vi "DetermineSetChosen.vi"(6 "Settings":T2={"Name of test"="", "Date"=timestamp(0 s since 1904-01-01), "Location"="", "Template"="", "Soundcard"="", "resolution"=32, "Sampling rate"=48000, "Ch1 Gain "=25.0, "Ch2 Gain"=10.0, "Sample time (s)"=0.3, "Pre-trigger (s)"=0.01, "Hammer Threshold"=10.0, "Positions"=12, "Taps/Position"=5, "Set Names"="", "Freq resolution"=10.0, "Hammer cutoff"=0.0, "Mic cutoff"=0.0, "Double bounce "=0.0, "Hammer Cal"=10.0, "dB Offset"=0.0, "Accel Cal"=10.0, "Vibrometer Cal"=0.0, "Mic Cal"=0.0, "Output"=2, "Voltage Cal"=1.0, "Vibrometer Port"="ASRL27::INSTR", "Range"=4, "High Pass"=2, "Bandwidth"=4, "X Range"=[], "Y Range"=[], "dB Spread"=0.0, "Trigger"=0, "Ch_1"=25, "Ch_2"=25, "flip?"=FALSE, "60Hz"=FALSE, "Time offset"=0.0, "Piezo Cal"=1.0, "Default Notes"=""} {"Ch_2" min=1 step=1; "Ch_1" min=1 max=100 step=1; "Trigger" items=["Hammer (force)", "Self-tap", "Spacebar"]; "Bandwidth" items=["1 kHz"=1, "5 kHz"=5, "10 kHz"=10, "25 kHz"=25, "50 kHz"=50, "100 kHz"=100]; "High Pass" items=["Off", "13 Hz", "104 Hz"]; "Range" items=["10 mm/s"=1, "20 mm/s"=2, "50 mm/s"=5, "100 mm/s"=10, "200 mm/s"=20, "500 mm/s"=50, "1 m/s"=100, "2 m/s"=200]; "Output" items=["Accelerometer", "Speed (from acceleration)", "Microphone", "Vibrometer", "Piezo"]; "Voltage Cal" format="%#_13g"; "Ch2 Gain" format="%#_13g"; "Ch1 Gain" format="%#_13g"; "Double bounce" min=0.0; "Mic cutoff" min=0.0 format="%#_4g"; "Hammer cutoff" min=0.0 format="%#_4g"; "Freq resolution" min=0.0; "Pre-trigger (s)" format="%#_13g"; "Date" format="%<%H:%M\n%d/%m/%y>T"; "resolution" items=["16 bit"=16, "24 bit"=24, "32 bit"=32]; "Sampling rate" items=["22050 samp/s"=22050, "44100 samp/s"=44100, "48000 samp/s"=48000]}, 9 "Bounds":T1, 11 "Mouse":T3) -> (1 "Queue Task":string, 3 "appended path":path)   [LabVIEW 2022 SP3]
uses:
  <vilib>/Utility/miscctls.llb/LVMouseTypeDef.ctl
  PreferencesControl.ctl
  <vilib>/Utility/miscctls.llb/LVBoundsTypeDef.ctl
  Mic/Mic_Global.vi
panel:
  in  "Cancel":bool
  in  "Just":bool
  in  "Subsequent":bool
  out "resulting string":string
  # "Hz"
  # "dB"
  # "dB"
  # "sec"
  # "sec"
  # "mV/Pa"
  # "mV/m/s2"
  # "mV/mm/s"
  # "V/N"
  # "sec"
  # "sec"
  # "mV/N"
  # "a.u."
  # "a.u."
  # "sec"
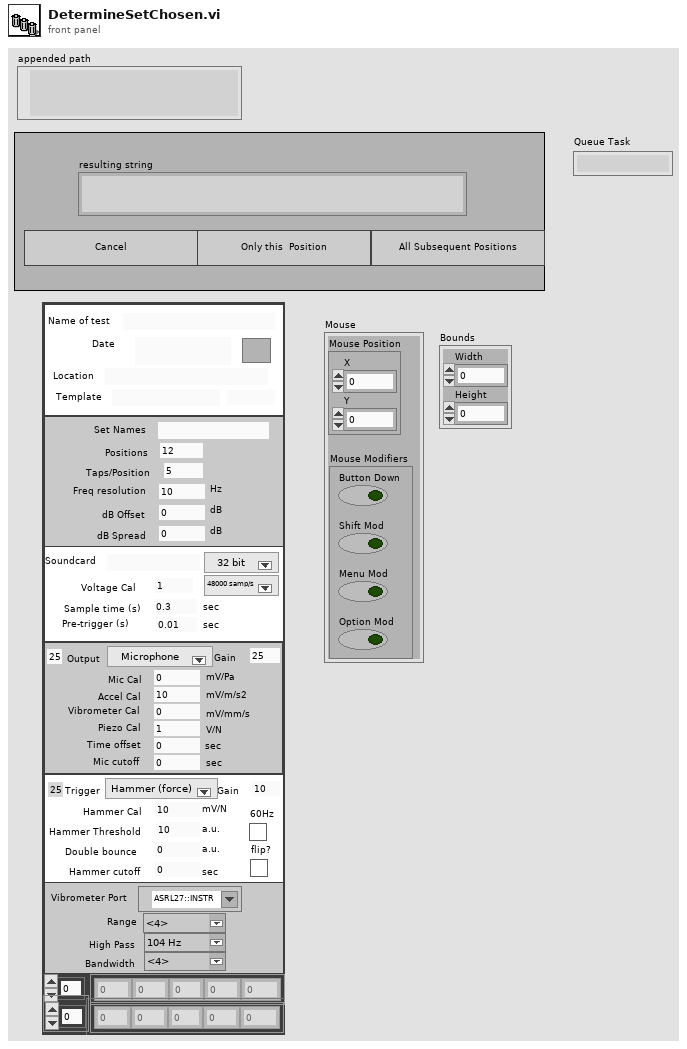
[diagram p1: front panel]
types:
  T1 = typedef "LVBoundsTypeDef.ctl" = cluster{"Width":u32, "Height":u32}
  T2 = typedef "PreferencesControl.ctl" = cluster{"Name of test":string, "Date":timestamp, "Location":string, "Template":string, "Soundcard":string, "resolution":u16, "Sampling rate":u16, "Ch1 Gain ":dbl, "Ch2 Gain":dbl, "Sample time (s)":dbl, "Pre-trigger (s)":dbl, "Hammer Threshold":dbl, "Positions":i16, "Taps/Position":i16, "Set Names":string, "Freq resolution":dbl, "Hammer cutoff":dbl, "Mic cutoff":dbl, "Double bounce ":dbl, "Hammer Cal":dbl, "dB Offset":dbl, "Accel Cal":dbl, "Vibrometer Cal":dbl, "Mic Cal":dbl, "Output":u16, "Voltage Cal":dbl, "Vibrometer Port":refnum<visa-resource-name>, "Range":u16, "High Pass":u16, "Bandwidth":u16, "X Range":cluster{"Minimum":dbl, "Maximum":dbl, "Increment":dbl, "Minor Increment":dbl, "Start":dbl}[], "Y Range":cluster{"Minimum":dbl, "Maximum":dbl, "Increment":dbl, "Minor Increment":dbl, "Start":dbl}[], "dB Spread":dbl, "Trigger":u16, "Ch_1":u8, "Ch_2":u8, "flip?":bool, "60Hz":bool, "Time offset":dbl, "Piezo Cal":dbl, "Default Notes":string}
  T3 = typedef "LVMouseTypeDef.ctl" = cluster{"Mouse Position":cluster{"X":i32, "Y":i32}, "Mouse Modifiers":cluster{"Button Down":bool, "Shift Mod":bool, "Menu Mod":bool, "Option Mod":bool}}
  T4 = cluster{"left":i16, "top":i16, "right":i16, "bottom":i16}[]
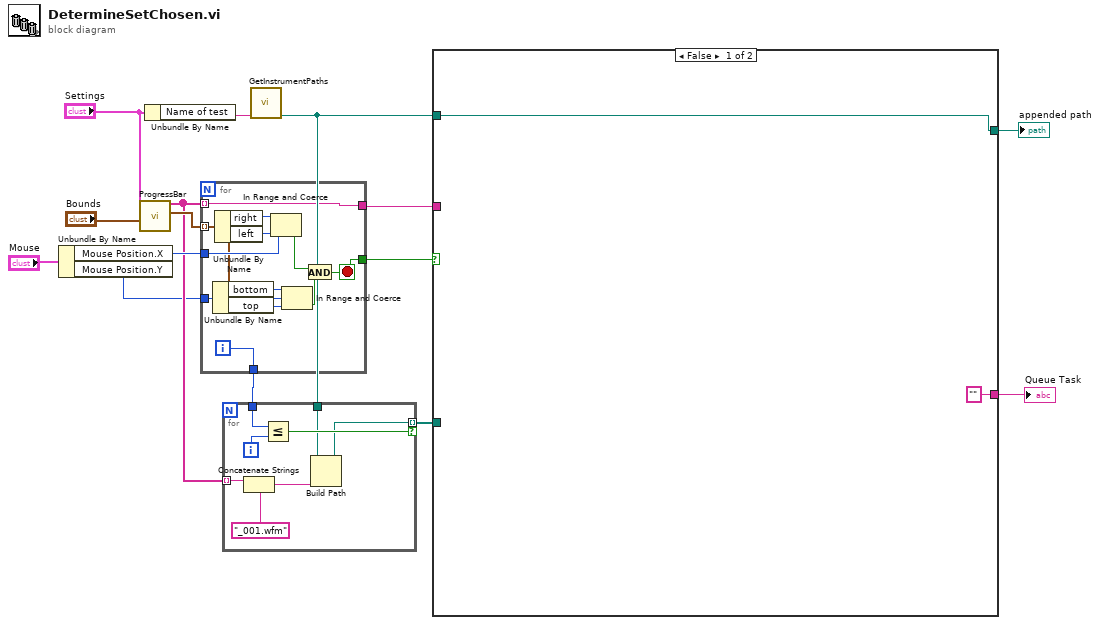
[diagram p0: block diagram]
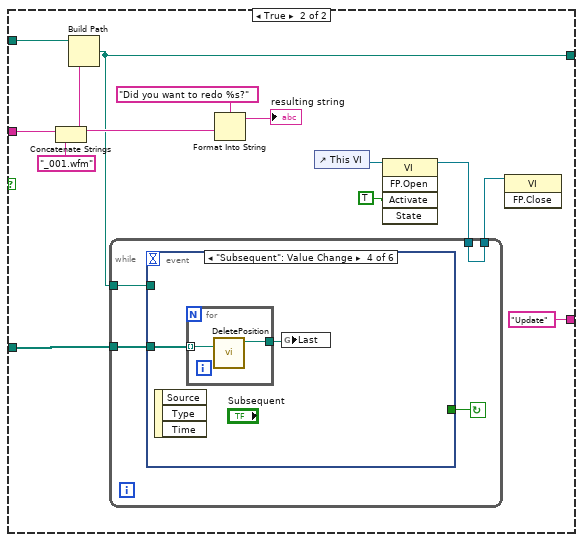
[diagram p2: hidden frame]
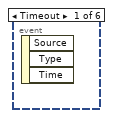
[diagram p3: hidden frame]
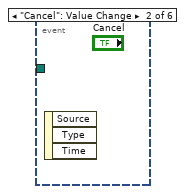
[diagram p4: hidden frame]
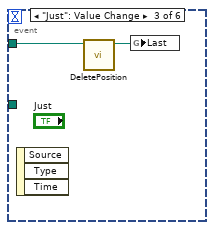
[diagram p5: hidden frame]
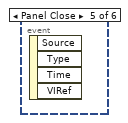
[diagram p6: hidden frame]
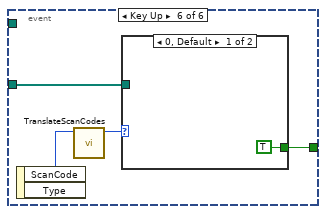
[diagram p7: hidden frame]
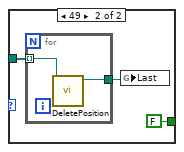
[diagram p8: hidden frame]
diagram:
  n1 = Unbundle By Name("Mouse") -> ("Mouse Position.X"=w15:i32, "Mouse Position.Y"=w3:i32)
  n2 = call "ProgressBar.vi"("Bounds"="Bounds", "Settings"="Settings") -> ("files"=w9:string[], "positions"=w14:T4)  [unwired: 7 in, 1 out]
  n3 = Unbundle By Name("Settings") -> ("Name of test"=w12:string)
  n4 = for {
    tunnel: w14 -> [w22] mode=indexing
    tunnel: w15 -> [w25]
    tunnel: [w24] -> w10
    tunnel: w9 -> [w24] mode=indexing
    tunnel: [w23] -> w8
    tunnel: w3 -> [w19]
    tunnel: [w16] -> w1
    i -> [w23]
    stop <- w16 stop-if-true
    n5 = Unbundle By Name(w22) -> ("bottom"=w21:i16, "top"=w20:i16)
    n6 = Unbundle By Name(w22) -> ("right"=w26:i16, "left"=w27:i16)
    n7 = In Range and Coerce(upper limit=w26, x=w25, lower limit=w27) -> (In Range?=w17:bool)  [unwired: 1 out]
    n8 = In Range and Coerce(upper limit=w21, x=w19, lower limit=w20) -> (In Range?=w18:bool)  [unwired: 1 out]
    n9 = And(x=w17, y=w18) -> (x .and. y?=w16:bool)
  }
  n10 = call "GetInstrumentPaths.vi"("Instrument"=w12) -> ("Path To Raw Folder"=w7:path)  [unwired: 6 in, 4 out]
  n11 = for {
    tunnel: w9 -> [w30] mode=indexing
    tunnel: w8 -> [w35]
    tunnel: [w28] -> w6 mode=indexing if=w33
    tunnel: w7 -> [w29]
    i -> [w34]
    n12 = Concatenate Strings(w30, "_001.wfm" ("string")) -> (w32:string)
    n13 = Less Or Equal?(x=w35, y=w34) -> (x <= y?=w33:bool)
    n14 = Build Path(base path=w29, name or relative path=w32) -> (appended path=w28:path)
  }
  n15 = case shown="False" w1 {
    tunnel: w10 -> [_ w47]
    tunnel: w7 -> [w37 w46]
    tunnel: w6 -> [_ w45]
    tunnel: [w37 w44] -> w5
    tunnel: ["" ("Queue Task") "Update" ("Queue Task")] -> w4
    frame False {
    }
    frame True {
      n16 = Concatenate Strings(w47, "_001.wfm" ("string")) -> (w49:string)
      n17 = Build Path(base path=w46, name or relative path=w49) -> (appended path=w44:path)
      n18 = Format Into String(format string="Did you want to redo %s?", w47) -> (resulting string=→"resulting string":string)  [unwired: 2 in, 1 out]
      n19 = control-ref of="This VI"() -> (w42:refnum<vi>)
      n20 = invoke class="VI" method="FP.Open"(reference=w42, "Activate"=TRUE ("Activate?")) -> (reference out=w39:refnum<vi>)  [unwired: 3 in, 4 out]
      n21 = while {
        tunnel: w44 -> [w54]
        tunnel: w45 -> [w53]
        tunnel: [w51] -> w40
        tunnel: w39 -> [w51]
        stop <- w52 continue-if-true
        n22 = event shown="[3] \"Subsequent\": Value Change" {
          selector: _ -> [_ _ _ _ _ _]
          dyn-events: _ -> [_ _ _ _ _ _]
          timeout: _ -> [_ _ _ _ _ _]
          tunnel: w54 -> [_ _ w55 _ _ _]
          tunnel: w53 -> [_ _ _ w58 _ w62]
          tunnel: [_ _ _ _ _ w61] -> w52
          event Timeout {
            n23 = event-data() -> ()  [unwired: 1 in, 3 out]
          }
          event "Cancel": Value Change {
            n24 = event-data() -> ()  [unwired: 1 in, 3 out]
          }
          event "Just": Value Change {
            n25 = event-data() -> ()  [unwired: 1 in, 3 out]
            n26 = call "DeletePosition.vi"("last"=w55) -> ("Last Data Set"=w56:path)  [unwired: 9 in, 1 out]
            n27 = global write "Mic_Global.vi" "Last"(w56) -> ()
          }
          event "Subsequent": Value Change {
            n28 = event-data() -> ()  [unwired: 1 in, 3 out]
            n29 = for {
              tunnel: w58 -> [w60] mode=indexing
              tunnel: [w59] -> w57
              n30 = call "DeletePosition.vi"("last"=w60) -> ("Last Data Set"=w59:path)  [unwired: 9 in, 1 out]
            }
            n31 = global write "Mic_Global.vi" "Last"(w57) -> ()
          }
          event Panel Close {
            n32 = event-data() -> ()  [unwired: 1 in, 4 out]
          }
          event Key Up {
            n33 = event-data() -> ("ScanCode"=w63:i16)  [unwired: 1 in, 1 out]
            n34 = call "TranslateScanCodes.vi"("ScanCode in"=w63) -> ("ScanCode out"=w64:i16)  [unwired: 10 in]
            n35 = case shown="0, Default" w64 {
              tunnel: w62 -> [_ w67]
              tunnel: [TRUE FALSE] -> w61
              frame 0, Default {
              }
              frame 49 {
                n36 = for {
                  tunnel: [w70] -> w68
                  tunnel: w67 -> [w69] mode=indexing
                  n37 = call "DeletePosition.vi"("last"=w69) -> ("Last Data Set"=w70:path)  [unwired: 9 in, 1 out]
                }
                n38 = global write "Mic_Global.vi" "Last"(w68) -> ()
              }
            }
          }
        }
      }
      n39 = invoke class="VI" method="FP.Close"(reference=w40) -> ()  [unwired: 2 in, 3 out]
    }
  }
  "appended path" <- w5
  "Queue Task" <- w4
